vi "GetStateData.vi"(8 "error in (no error)":errorcluster, 11 "UpstreamMsgParent in":refnum<class "UpstreamMsgParent.lvclass">) -> (0 "error out":errorcluster, 1 "Data":string, 2 "State":string, 3 "UpstreamMsgParent out":refnum<class "UpstreamMsgParent.lvclass">)   [LabVIEW 2020, in "UpstreamMsg.lvlib" / "UpstreamMsgParent.lvclass"]
uses:
  UpstreamMsgParent/UpstreamMsgParent.lvclass
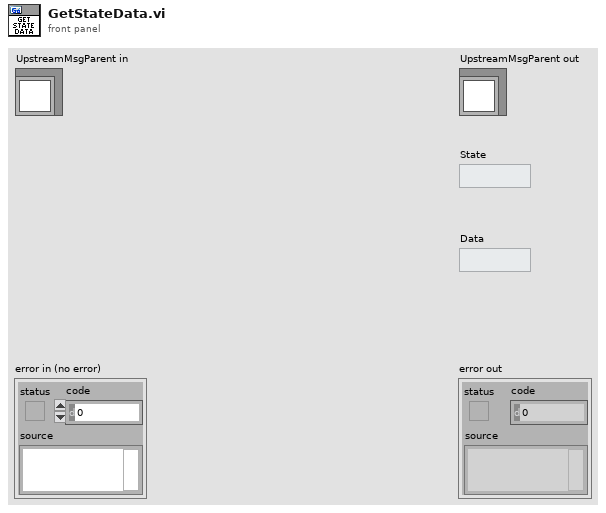
[diagram p1: front panel]
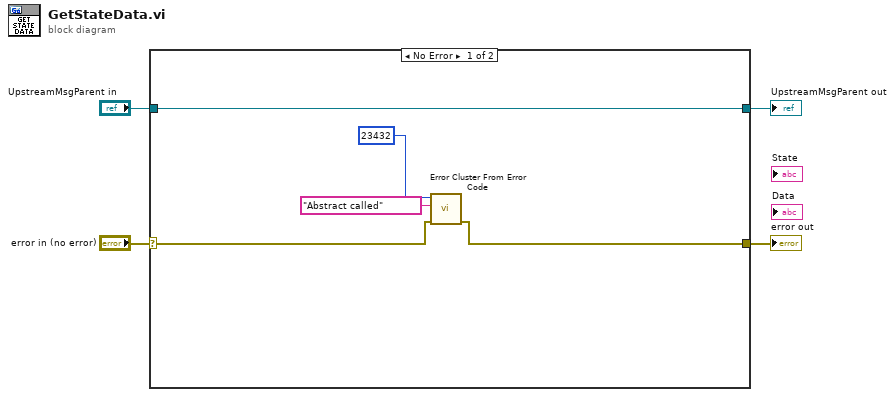
[diagram p0: block diagram]
diagram:
  n1 = case shown="No Error" "error in (no error)" {
    selector: "error in (no error)" -> [w8 w11]
    tunnel: [w7 w11] -> w3
    tunnel: [w9 w10] -> w1
    tunnel: "UpstreamMsgParent in" -> [w9 w10]
    frame No Error {
      n2 = call <vilib>:"Error Cluster From Error Code.vi"("error in (no error)"=w8, "error message (\"\")"="Abstract called" ("error message (\"\")"), "error code (0)"=23432) -> ("error out"=w7:errorcluster)  [unwired: 6 in]
    }
    frame Error {
    }
  }
  "error out" <- w3
  "UpstreamMsgParent out" <- w1
